vi "DischargeNoRecording.vi"() -> ()   [LabVIEW 2020]
uses:
  <instrlib>/NH Research Regenerative Test Series/Public/Configure/Output Safety.ctl
  <vilib>/DAQmx/read.llb/DAQmx Read (Analog 1D DBL NChan 1Samp).vi
  <instrlib>/NH Research Regenerative Test Series/Public/Data/Read (Ave Current).vi
  <instrlib>/NH Research Regenerative Test Series/Public/Data/Low Level/Fetch (Ave Voltage).vi
  <instrlib>/NH Research Regenerative Test Series/Public/Data/Low Level/Fetch (Ave True Power).vi
  <vilib>/DAQmx/miscellaneous.llb/DAQmx Fill In Error Info.vi
  <instrlib>/NH Research Regenerative Test Series/NH Research Regenerative Test Series.lvlib
panel:
  out "String 3":string
  out "Ave True Power (W) 3":dbl
  out "Ave Voltage (V) 3":dbl
  out "Ave Current (A) 3":dbl
  in  "Logical Instrument Number 3":u32=1
  in  "VISA resource name 3":refnum<visa-resource-name>
  out "String 2":string
  out "Ave True Power (W) 2":dbl
  out "Ave Voltage (V) 2":dbl
  out "Ave Current (A) 2":dbl
  in  "Logical Instrument Number 2":u32=1
  in  "VISA resource name 2":refnum<visa-resource-name>
  out "Temp2":dbl
  out "Temp1":dbl
  out "Task error out":errorcluster
  out "String":string
  in  "Output Safety":T1
  out "Filename Out":path
  in  "DAQmx Task Name":refnum<k21>
  out "Voltage Compare":dbl
  in  "Path":path
  in  "Voltage Cutoff":dbl
  out "Ave Current (A)":dbl
  out "Ave Voltage (V)":dbl
  out "Ave True Power (W)":dbl
  out "Status Byte Register":T2
  in  "Logical Instrument Number":u32=1
  in  "Current Setpoint (0 A)":dbl format="%#.6g"
  in  "Battery Detect Voltage (0V)":dbl format="%#.6g"
  in  "VISA resource name":refnum<visa-resource-name>
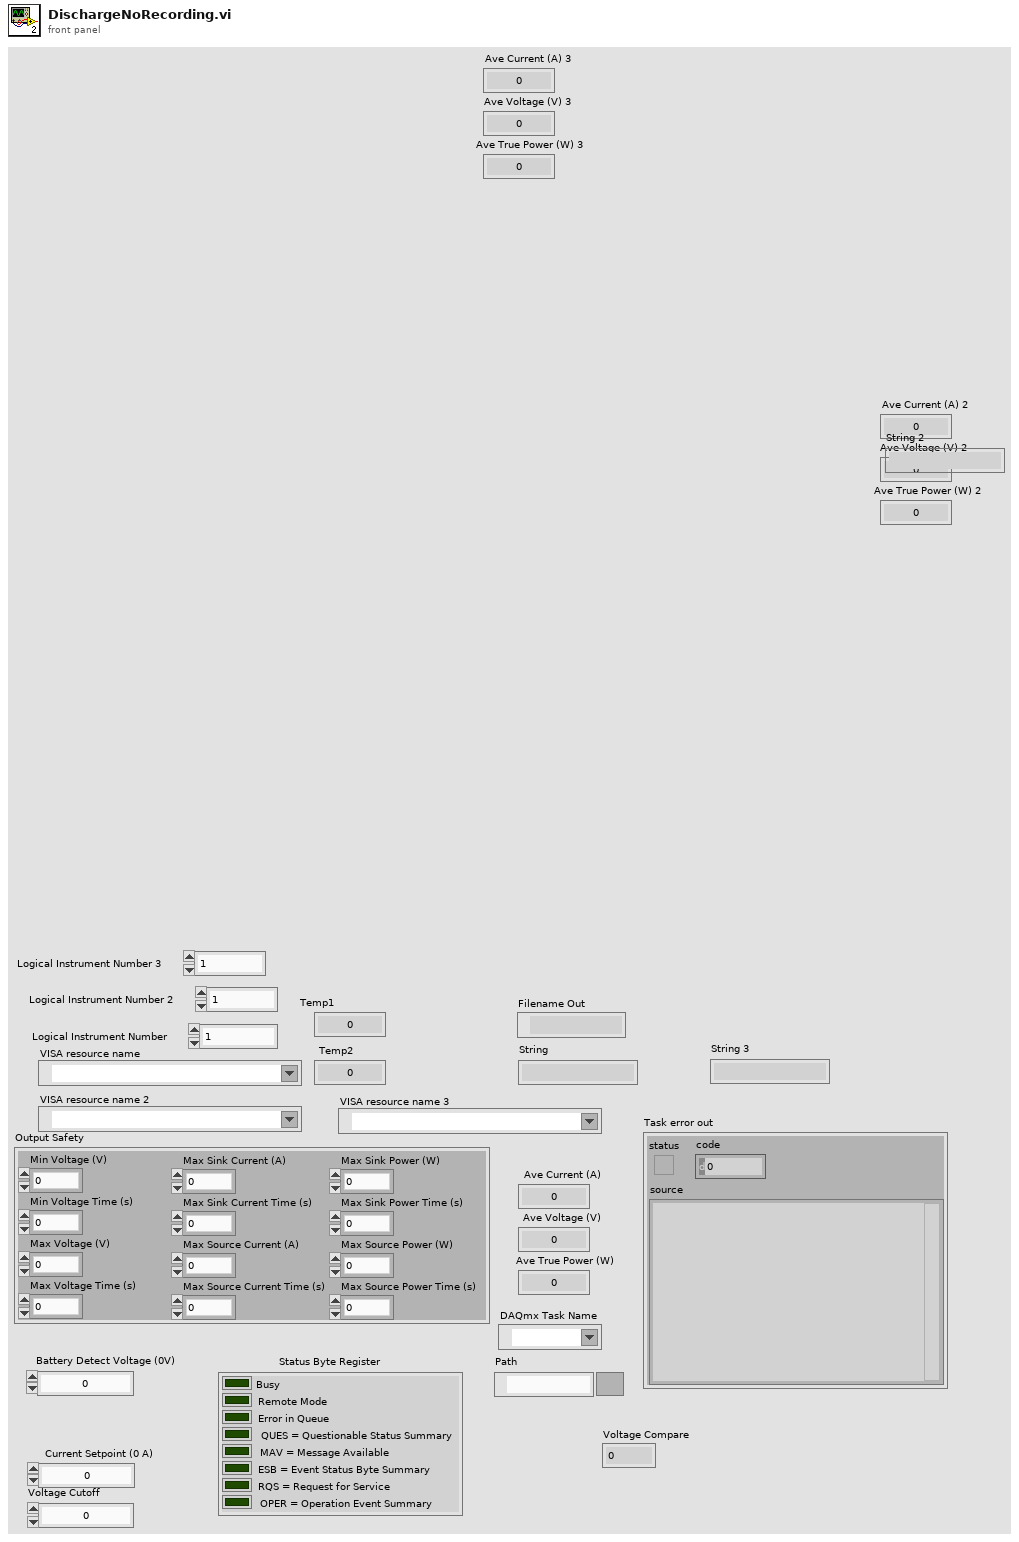
[diagram p1: front panel]
types:
  T1 = typedef "NH Research Regenerative Test Series.lvlib/Output Safety.ctl" = cluster{"Min Voltage (V)":dbl, "Min Voltage Time (s)":dbl, "Max Voltage (V)":dbl, "Max Voltage Time (s)":dbl, "Max Sink Current (A)":dbl, "Max Sink Current Time (s)":dbl, "Max Source Current (A)":dbl, "Max Source Current Time (s)":dbl, "Max Sink Power (W)":dbl, "Max Sink Power Time (s)":dbl, "Max Source Power (W)":dbl, "Max Source Power Time (s)":dbl}
  T2 = cluster{"Busy":bool, "Remote Mode":bool, "Error in Queue":bool, "QUES = Questionable Status Summary":bool, "MAV = Message Available":bool, "ESB = Event Status Byte Summary":bool, "RQS = Request for Service":bool, "OPER = Operation Event Summary":bool}
  T3 = cluster{"data[0]":dbl, "data[1]":dbl, "data[2]":dbl, "data[3]":dbl, "data[4]":dbl, "data[5]":dbl, "data[6]":dbl, "data[7]":dbl, "data[8]":dbl}
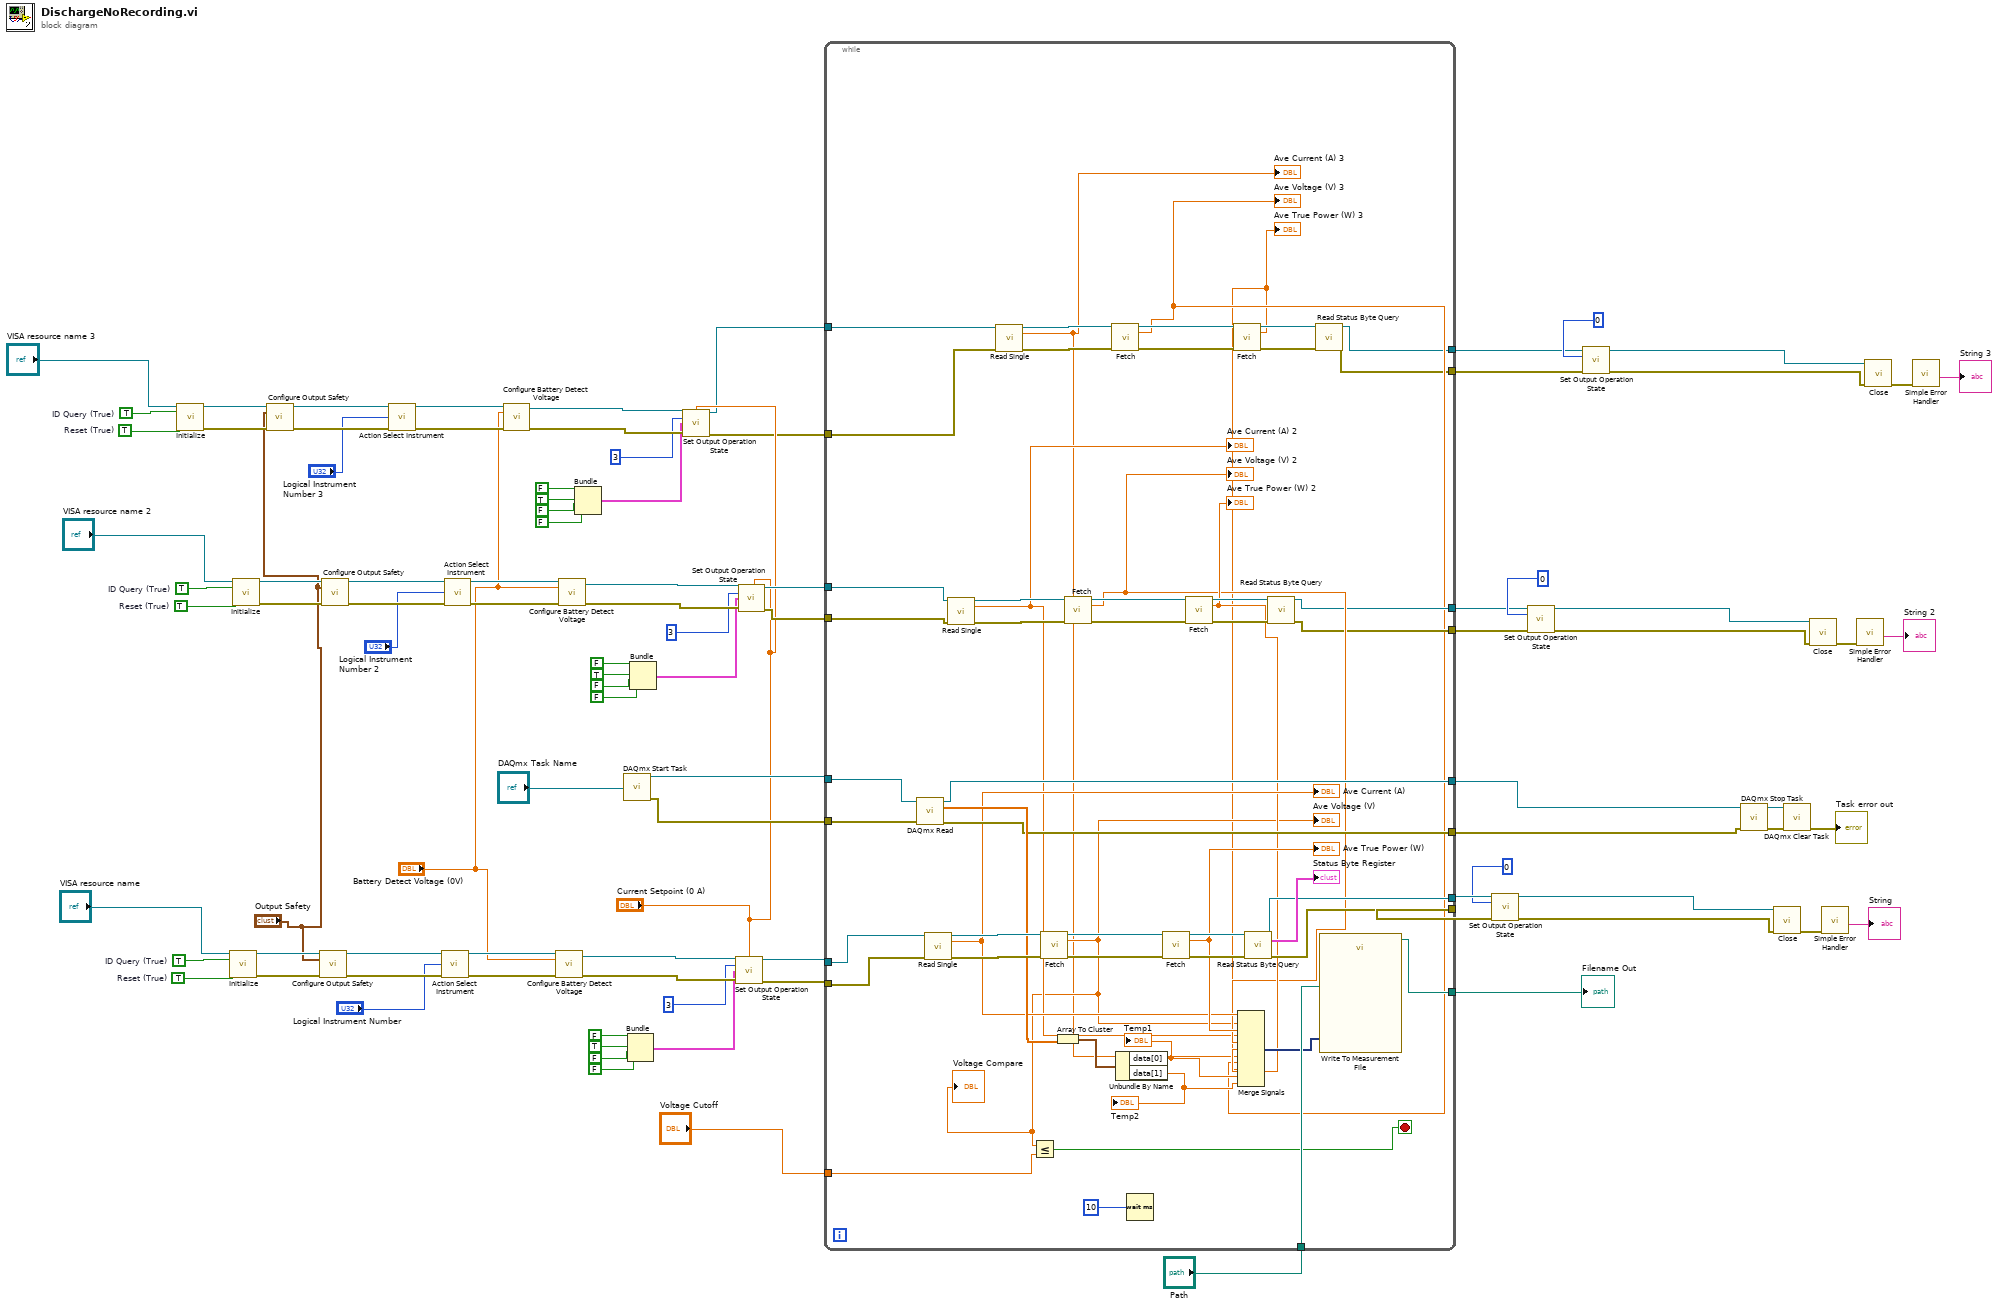
[diagram p0: block diagram]
diagram:
  w20 = TRUE  # ID Query (True)
  w19 = TRUE  # Reset (True)
  w48 = TRUE  # ID Query (True)
  w47 = TRUE  # Reset (True)
  w77 = TRUE  # ID Query (True)
  w76 = TRUE  # Reset (True)
  n1 = call <vilib>:"Initialize.vi"("VISA resource name"="VISA resource name 3", "ID Query (True)"=w20, "Reset (True)"=w19) -> ("VISA resource name out"=w18:refnum<visa-resource-name>, "error out"=w17:errorcluster)  [unwired: 11 in]
  n2 = call <vilib>:"Initialize.vi"("VISA resource name"="VISA resource name", "ID Query (True)"=w77, "Reset (True)"=w76) -> ("VISA resource name out"=w75:refnum<visa-resource-name>, "error out"=w74:errorcluster)  [unwired: 11 in]
  n3 = call <vilib>:"Initialize.vi"("VISA resource name"="VISA resource name 2", "ID Query (True)"=w48, "Reset (True)"=w47) -> ("VISA resource name out"=w46:refnum<visa-resource-name>, "error out"=w45:errorcluster)  [unwired: 11 in]
  n4 = call <vilib>:"Configure Output Safety.vi"("VISA resource name"=w18, "Output Safety"="Output Safety", "error in (no error)"=w17) -> ("VISA resource name out"=w15:refnum<visa-resource-name>, "error out"=w14:errorcluster)  [unwired: 11 in]
  n5 = call <vilib>:"Configure Output Safety.vi"("VISA resource name"=w75, "Output Safety"="Output Safety", "error in (no error)"=w74) -> ("VISA resource name out"=w72:refnum<visa-resource-name>, "error out"=w59:errorcluster)  [unwired: 11 in]
  n6 = call <vilib>:"Configure Output Safety.vi"("VISA resource name"=w46, "Output Safety"="Output Safety", "error in (no error)"=w45) -> ("VISA resource name out"=w43:refnum<visa-resource-name>, "error out"=w42:errorcluster)  [unwired: 11 in]
  n7 = call <instrlib>:"Action Select Instrument.vi"("VISA resource name"=w15, "Logical Instrument Number"="Logical Instrument Number 3", "error in (no error)"=w14) -> ("VISA resource name out"=w30:refnum<visa-resource-name>, "error out"=w29:errorcluster)  [unwired: 11 in]
  n8 = call <instrlib>:"Action Select Instrument.vi"("VISA resource name"=w72, "Logical Instrument Number"="Logical Instrument Number", "error in (no error)"=w59) -> ("VISA resource name out"=w95:refnum<visa-resource-name>, "error out"=w94:errorcluster)  [unwired: 11 in]
  n9 = call <instrlib>:"Action Select Instrument.vi"("VISA resource name"=w43, "Logical Instrument Number"="Logical Instrument Number 2", "error in (no error)"=w42) -> ("VISA resource name out"=w58:refnum<visa-resource-name>, "error out"=w57:errorcluster)  [unwired: 11 in]
  n10 = call <vilib>:"Configure Battery Detect Voltage.vi"("VISA resource name"=w30, "Battery Detect Voltage (0V)"="Battery Detect Voltage (0V)", "error in (no error)"=w29) -> ("VISA resource name out"=w28:refnum<visa-resource-name>, "error out"=w27:errorcluster)  [unwired: 11 in]
  n11 = call <vilib>:"Configure Battery Detect Voltage.vi"("VISA resource name"=w95, "Battery Detect Voltage (0V)"="Battery Detect Voltage (0V)", "error in (no error)"=w94) -> ("VISA resource name out"=w93:refnum<visa-resource-name>, "error out"=w92:errorcluster)  [unwired: 11 in]
  n12 = call <vilib>:"Configure Battery Detect Voltage.vi"("VISA resource name"=w58, "Battery Detect Voltage (0V)"="Battery Detect Voltage (0V)", "error in (no error)"=w57) -> ("VISA resource name out"=w56:refnum<visa-resource-name>, "error out"=w55:errorcluster)  [unwired: 11 in]
  n13 = Bundle(FALSE, TRUE, FALSE, FALSE) -> (w21:cluster{bool, bool, bool, bool})  [unwired: 1 in]
  n14 = call <vilib>:"DAQmx Start Task.vi"("task/channels in"="DAQmx Task Name") -> ("task out"=w70:refnum<k21>, "error out"=w60:errorcluster)  [unwired: 13 in]
  n15 = Bundle(FALSE, TRUE, FALSE, FALSE) -> (w81:cluster{bool, bool, bool, bool})  [unwired: 1 in]
  n16 = Bundle(FALSE, TRUE, FALSE, FALSE) -> (w49:cluster{bool, bool, bool, bool})  [unwired: 1 in]
  n17 = call <vilib>:"Set Output Operation State.vi"("VISA resource name"=w28, "Current Setpoint (0 A)"="Current Setpoint (0 A)", "Mode (0: Off)"=3, "Enable"=w21, "error in (no error)"=w27) -> ("VISA resource name out"=w9:refnum<visa-resource-name>, "error out"=w8:errorcluster)  [unwired: 9 in]
  n18 = call <vilib>:"Set Output Operation State.vi"("VISA resource name"=w93, "Current Setpoint (0 A)"="Current Setpoint (0 A)", "Mode (0: Off)"=3, "Enable"=w81, "error in (no error)"=w92) -> ("VISA resource name out"=w88:refnum<visa-resource-name>, "error out"=w87:errorcluster)  [unwired: 9 in]
  n19 = call <vilib>:"Set Output Operation State.vi"("VISA resource name"=w56, "Current Setpoint (0 A)"="Current Setpoint (0 A)", "Mode (0: Off)"=3, "Enable"=w49, "error in (no error)"=w55) -> ("VISA resource name out"=w39:refnum<visa-resource-name>, "error out"=w38:errorcluster)  [unwired: 9 in]
  n20 = while {
    tunnel: w88 -> [w143]
    tunnel: w87 -> [w142]
    tunnel: [w140] -> w91
    tunnel: [w139] -> w90
    tunnel: "Voltage Cutoff" -> [w127]
    tunnel: "Path" -> [w137]
    tunnel: w70 -> [w136]
    tunnel: [w132] -> w62
    tunnel: [w131] -> w61
    tunnel: w60 -> [w130]
    tunnel: [w129] -> w78
    tunnel: w39 -> [w115]
    tunnel: w38 -> [w114]
    tunnel: [w113] -> w32
    tunnel: [w112] -> w31
    tunnel: w9 -> [w104]
    tunnel: w8 -> [w103]
    tunnel: [w97] -> w2
    tunnel: [w96] -> w1
    stop <- w128 stop-if-true
    n21 = call-poly <vilib>:"DAQmx Read.vi"("task/channels in"=w136, "error in"=w130) -> ("task out"=w132:refnum<k21>, "data"=w135:dbl[], "error out"=w131:errorcluster)  [unwired: 11 in]
    n22 = call-poly <instrlib>:"Read Single.vi"("VISA resource name"=w143, "error in (no error)"=w142) -> ("VISA resource name out"=w148:refnum<visa-resource-name>, "Ave Current (A)"=w126:dbl, "error out"=w149:errorcluster)  [unwired: 11 in]
    "Ave Current (A)" <- w126
    n23 = call-poly <instrlib>:"Read Single.vi"("VISA resource name"=w115, "error in (no error)"=w114) -> ("VISA resource name out"=w123:refnum<visa-resource-name>, "Ave Current (A)"=w116:dbl, "error out"=w124:errorcluster)  [unwired: 11 in]
    "Ave Current (A) 2" <- w116
    n24 = call-poly <instrlib>:"Read Single.vi"("VISA resource name"=w104, "error in (no error)"=w103) -> ("VISA resource name out"=w109:refnum<visa-resource-name>, "Ave Current (A)"=w100:dbl, "error out"=w110:errorcluster)  [unwired: 11 in]
    "Ave Current (A) 3" <- w100
    n25 = call-poly <instrlib>:"Fetch.vi"("VISA resource name"=w148, "error in (no error)"=w149) -> ("VISA resource name out"=w147:refnum<visa-resource-name>, "Ave Voltage (V)"=w111:dbl, "error out"=w146:errorcluster)  [unwired: 11 in]
    "Ave Voltage (V)" <- w111
    "Voltage Compare" <- w111
    n26 = Less Or Equal?(x=w111, y=w127) -> (x <= y?=w128:bool)
    n27 = Array To Cluster(array=w135) -> (cluster=w134:T3)
    n28 = call-poly <instrlib>:"Fetch.vi"("VISA resource name"=w123, "error in (no error)"=w124) -> ("VISA resource name out"=w122:refnum<visa-resource-name>, "Ave Voltage (V)"=w117:dbl, "error out"=w121:errorcluster)  [unwired: 11 in]
    "Ave Voltage (V) 2" <- w117
    n29 = call-poly <instrlib>:"Fetch.vi"("VISA resource name"=w109, "error in (no error)"=w110) -> ("VISA resource name out"=w108:refnum<visa-resource-name>, "Ave Voltage (V)"=w99:dbl, "error out"=w107:errorcluster)  [unwired: 11 in]
    "Ave Voltage (V) 3" <- w99
    n30 = Unbundle By Name(w134) -> ("data[0]"=w102:dbl, "data[1]"=w101:dbl)
    "Temp1" <- w102
    "Temp2" <- w101
    n31 = Wait (ms)(milliseconds to wait=10) -> ()  [unwired: 1 out]
    n32 = call-poly <instrlib>:"Fetch.vi"("VISA resource name"=w147, "error in (no error)"=w146) -> ("VISA resource name out"=w145:refnum<visa-resource-name>, "Ave True Power (W)"=w138:dbl, "error out"=w144:errorcluster)  [unwired: 11 in]
    "Ave True Power (W)" <- w138
    n33 = call-poly <instrlib>:"Fetch.vi"("VISA resource name"=w122, "error in (no error)"=w121) -> ("VISA resource name out"=w120:refnum<visa-resource-name>, "Ave True Power (W)"=w118:dbl, "error out"=w119:errorcluster)  [unwired: 11 in]
    "Ave True Power (W) 2" <- w118
    n34 = call-poly <instrlib>:"Fetch.vi"("VISA resource name"=w108, "error in (no error)"=w107) -> ("VISA resource name out"=w106:refnum<visa-resource-name>, "Ave True Power (W)"=w98:dbl, "error out"=w105:errorcluster)  [unwired: 11 in]
    "Ave True Power (W) 3" <- w98
    n35 = Merge Signals "Merge Signals"(w126, w111, w138, w116, w117, w118, w100, w99, w98, w102, w101) -> (w133:dynamicdata)
    n36 = call <instrlib>:"Read Status Byte Query.vi"("VISA resource name"=w145, "error in (no error)"=w144) -> ("VISA resource name out"=w140:refnum<visa-resource-name>, "Status Byte Register"=→"Status Byte Register":T2, "error out"=w139:errorcluster)  [unwired: 11 in]
    n37 = call <instrlib>:"Read Status Byte Query.vi"("VISA resource name"=w120, "error in (no error)"=w119) -> ("VISA resource name out"=w113:refnum<visa-resource-name>, "error out"=w112:errorcluster)  [unwired: 11 in, 1 out]
    n38 = call <instrlib>:"Read Status Byte Query.vi"("VISA resource name"=w106, "error in (no error)"=w105) -> ("VISA resource name out"=w97:refnum<visa-resource-name>, "error out"=w96:errorcluster)  [unwired: 11 in, 1 out]
    n39 = call "Write To Measurement File"("Signals"=w133, "Filename"=w137) -> ("Filename Out"=w129:path)  [unwired: 15 in, 2 out]
  }
  "Filename Out" <- w78
  n40 = call <vilib>:"Set Output Operation State.vi"("VISA resource name"=w91, "Mode (0: Off)"=0, "error in (no error)"=w90) -> ("VISA resource name out"=w64:refnum<visa-resource-name>, "error out"=w63:errorcluster)  [unwired: 11 in]
  n41 = call <vilib>:"Set Output Operation State.vi"("VISA resource name"=w32, "Mode (0: Off)"=0, "error in (no error)"=w31) -> ("VISA resource name out"=w34:refnum<visa-resource-name>, "error out"=w33:errorcluster)  [unwired: 11 in]
  n42 = call <vilib>:"Set Output Operation State.vi"("VISA resource name"=w2, "Mode (0: Off)"=0, "error in (no error)"=w1) -> ("VISA resource name out"=w4:refnum<visa-resource-name>, "error out"=w3:errorcluster)  [unwired: 11 in]
  n43 = call <vilib>:"DAQmx Stop Task.vi"("task/channels in"=w62, "error in"=w61) -> ("task out"=w68:refnum<k21>, "error out"=w67:errorcluster)  [unwired: 12 in]
  n44 = call <instrlib>:"Close.vi"("VISA resource name"=w64, "error in (no error)"=w63) -> ("error out"=w65:errorcluster)  [unwired: 13 in]
  n45 = call <vilib>:"DAQmx Clear Task.vi"("task in"=w68, "error in"=w67) -> ("error out"=→"Task error out":errorcluster)  [unwired: 13 in]
  n46 = call <instrlib>:"Close.vi"("VISA resource name"=w34, "error in (no error)"=w33) -> ("error out"=w35:errorcluster)  [unwired: 13 in]
  n47 = call <vilib>:"Simple Error Handler.vi"("error in (no error)"=w65) -> ("source out"=→"String":string)  [unwired: 4 in, 4 out]
  n48 = call <vilib>:"Simple Error Handler.vi"("error in (no error)"=w35) -> ("source out"=→"String 2":string)  [unwired: 4 in, 4 out]
  n49 = call <instrlib>:"Close.vi"("VISA resource name"=w4, "error in (no error)"=w3) -> ("error out"=w5:errorcluster)  [unwired: 13 in]
  n50 = call <vilib>:"Simple Error Handler.vi"("error in (no error)"=w5) -> ("source out"=→"String 3":string)  [unwired: 4 in, 4 out]
